vi "Initialise POI and Miniscan selector arrays.vi"(8 "error in (no error)":errorcluster) -> (0 "error out":errorcluster, 1 "[ROI vis]":T1 caption="[POI#]" {"ROI number" min=1 format="ROI %.0f"}, 4 "Number of POI":i32, 6 "Number of Miniscans":i32)   [LabVIEW 2013]
uses:
  Typedefs/ROI selector array-ROI vis.ctl
  xcontrol/Interface VIs/Interface typedefs/Interface-ROI selection cluster.ctl
  Typedefs/ROI ID Enum.ctl
  Typedefs/Get-Set-Clear Control.ctl
  Global variables/gl_Functional Imaging-Global variables.vi
panel:
  # "<-- used duting initialisation only"
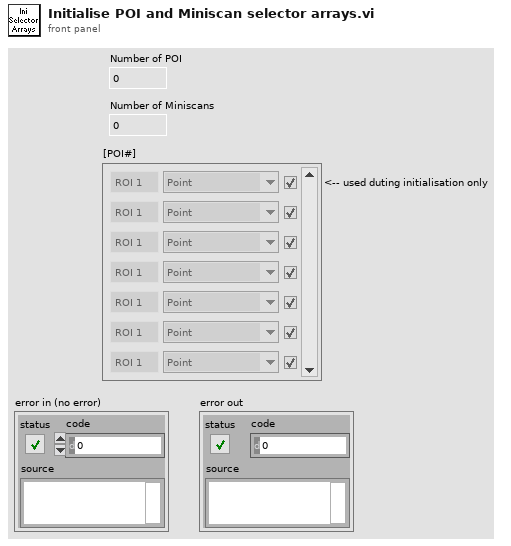
[diagram p1: front panel]
types:
  T1 = typedef "ROI selector array-ROI vis.ctl" = T2[]
  T2 = typedef "Interface-ROI selection cluster.ctl" = cluster{"ROI number":i32, "ROI ID":T3, "Visibility":bool}
  T3 = typedef "ROI ID Enum.ctl" = enum16{"Point", "MiniScan", "Comp. MiniScan", "Rectangle", "Comp. volume", "Arb. plane point"}
  T4 = typedef "Get-Set-Clear Control.ctl" = enum16{"Get", "Set", "Clear"}
  T5 = typedef "ROI indexes by type.ctl" = cluster{"Indexes of POI":i32[], "Indexes of Miniscans":i32[], "Indexes of? (Provisional)":i32[]}
  T6 = typedef "Functional Imging UI Refs.ctl" = cluster{"Menu ref":refnum<k9>, "Image control":refnum<vi>, "VI ref":refnum<vi>, "XGrapher":refnum<vi>, "Smoothing":refnum<vi>, "POI Averaging":refnum<vi>, "Normalize":refnum<vi>, "POI data points in each trial":refnum<vi>, "Channel":refnum<vi>, "Experiment data folder path":refnum<vi>, "[ROI vis]":refnum<vi>, "[Groups] visbl":T7, "Group Name":refnum<vi>, "POI index":refnum<vi>, "Trial No.":refnum<vi>, "Intensity Zoom":refnum<vi>, "Trial Cursor Enabled":refnum<vi>, "Number of Trials (ind 1)":refnum<vi>, "Number of Trials (ind 2)":refnum<vi>, "MiniScans Available":refnum<vi>, "POI Available":refnum<vi>, "Defer graph updates":refnum<vi>, "Waveform selector":refnum<vi>, "#of selected POI":refnum<vi>, "#of selected MiniScans":refnum<vi>, "#of selected groups":refnum<vi>, "Max Z-Projection":refnum<vi>, "Z-Plane Selector":refnum<vi>, "Index of miniscan point to visualise":refnum<vi>, "ROI vis. mode":refnum<vi>, "Total # of points":refnum<vi>, "Index of group clicked on":refnum<vi>, "Pane 1":refnum<vi>, "Pane 2":refnum<vi>, "Pane 3":refnum<vi>, "Pane 4":refnum<vi>, "Pane 5":refnum<vi>, "Pane 6":refnum<vi>, "Deselect all ROI":refnum<vi>, "Deselect all groups":refnum<vi>}
  T7 = typedef "Groups array referecne.ctl" = refnum<vi>
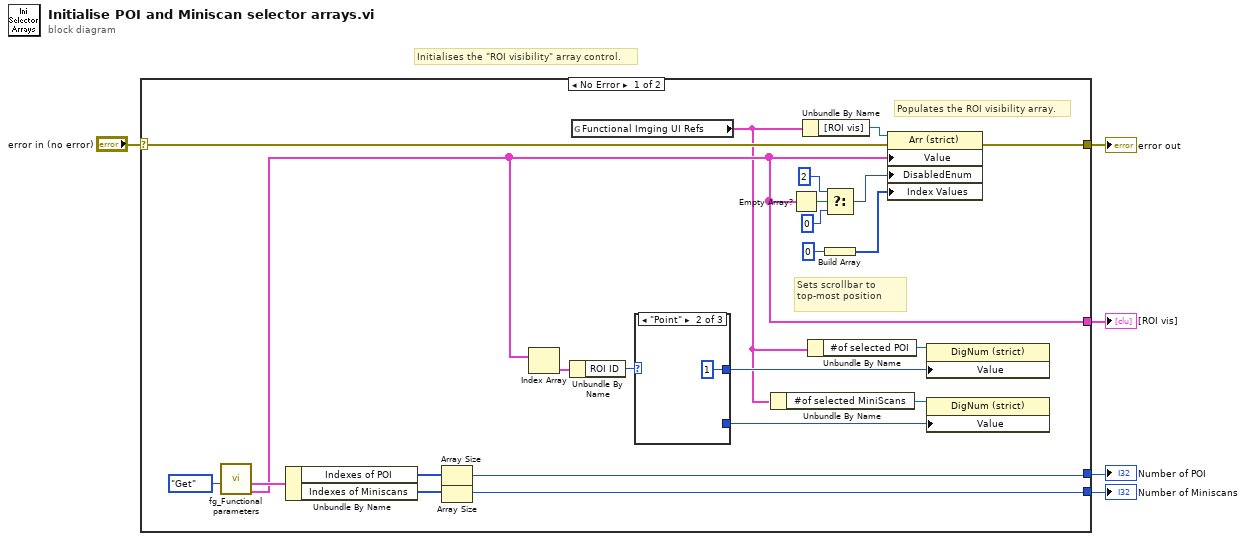
[diagram p0: block diagram]
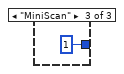
[diagram p3: hidden frame]
diagram:
  # "Initialises the \"ROI visibility\" array control."
  n1 = case shown="No Error" "error in (no error)" {
    selector: "error in (no error)" -> [w25 w31]
    tunnel: [w13 _] -> w5
    tunnel: [w18 w31] -> w3
    tunnel: [w21 _] -> w2
    tunnel: [w20 _] -> w1
    frame No Error {
      # "Populates the ROI visibility array."
      # "Sets scrollbar to top-most position"
      n2 = call "fg_Functional parameters.vi"("Function"=Get-Set-Clear_Control."Get") -> ("[ROI vis]"=w13:T1, "ROI indexes by type"=w23:T5)  [unwired: 7 in, 2 out]
      n3 = Unbundle By Name(w23) -> ("Indexes of POI"=w24:i32[], "Indexes of Miniscans"=w7:i32[])
      n4 = Array Size(array=w24) -> (size(s)=w21:i32)
      n5 = Array Size(array=w7) -> (size(s)=w20:i32)
      n6 = Index Array(array=w13) -> (element=w12:T2)  [unwired: 1 in]
      n7 = Unbundle By Name(w12) -> ("ROI ID"=w10:T3)
      n8 = global read "gl_Functional Imaging-Global variables.vi" "Functional Imging UI Refs"() -> (w6:T6)
      n9 = case shown="\"Point\"" w10 {
        tunnel: [_ 1 ("Value") _] -> w9
        tunnel: [_ _ 1 ("Value")] -> w8
        frame Default {
        }
        frame "Point" {
        }
        frame "MiniScan" {
        }
      }
      n10 = Unbundle By Name(w6) -> ("#of selected MiniScans"=w19:refnum<vi>)
      n11 = Empty Array?(array=w13) -> (empty?=w27:bool)
      n12 = Unbundle By Name(w6) -> ("[ROI vis]"=w28:refnum<vi>)
      n13 = Unbundle By Name(w6) -> ("#of selected POI"=w11:refnum<vi>)
      n14 = Select(t=2, s=w27, f=0) -> (s? t:f=w26:i32)
      n15 = Build Array(u32 0) -> (w14:u32[])
      n16 = property class="Arr (strict)"(reference=w28, error in=w25, "Value"=w13, "DisabledEnum"=w26, "Index Values"=w14) -> (error out=w18:errorcluster)  [unwired: 1 out]
      n17 = property on="Property Node" class="DigNum (strict)"(reference=w11, "Value"=w9) -> ()  [unwired: 1 in, 2 out]
      n18 = property on="Property Node" class="DigNum (strict)"(reference=w19, "Value"=w8) -> ()  [unwired: 1 in, 2 out]
    }
    frame Error {
    }
  }
  "error out" <- w3
  "[ROI vis]" <- w5
  "Number of POI" <- w2
  "Number of Miniscans" <- w1
